vi "ExecuteFile.vi"(0 "File Name With Extension":string) -> ()   [LabVIEW 2015]
panel:
  out "error out":errorcluster
  out "File Contents":string
  out "Lines":string[](array[string])
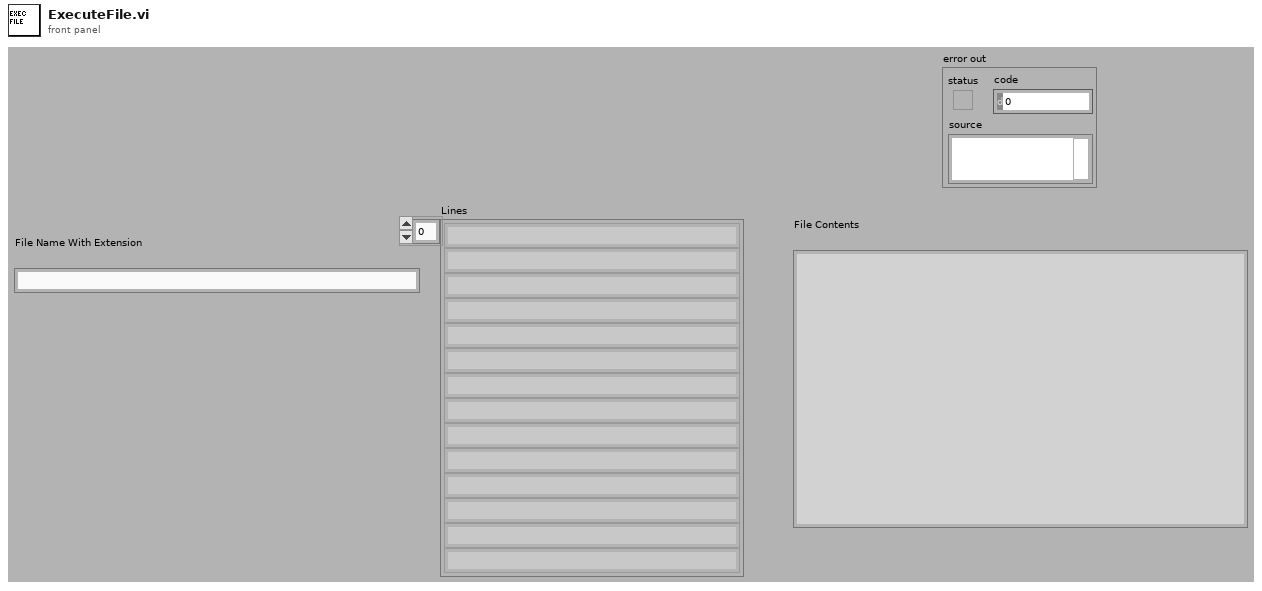
[diagram p1: front panel]
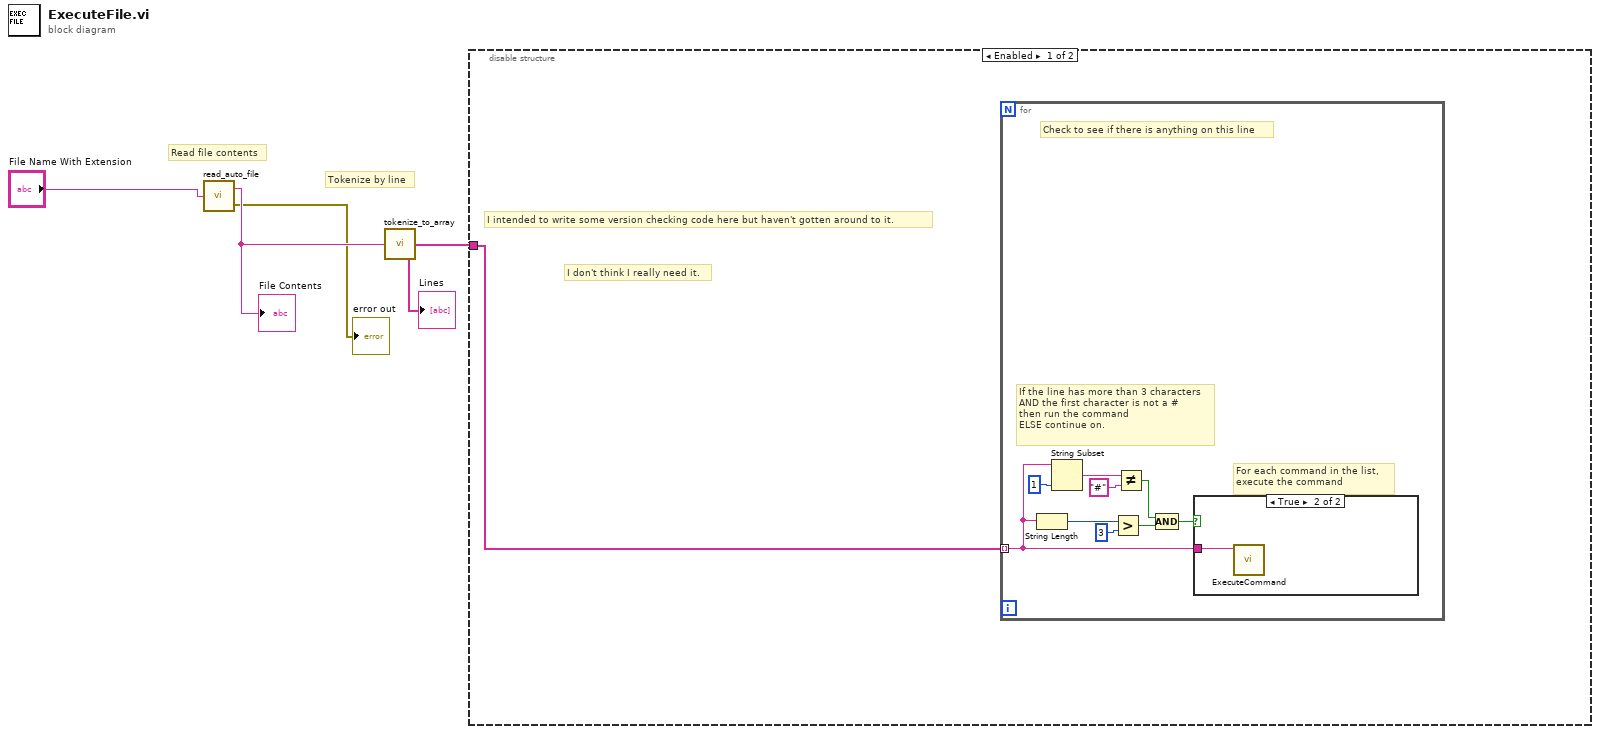
[diagram p0: block diagram]
diagram:
  # "Tokenize by line"
  # "Read file contents"
  n1 = call "read_auto_file.vi"("File Name With Extension"="File Name With Extension") -> ("File Contents"=w4:string, "error out"=→"error out":errorcluster)
  "File Contents" <- w4
  n2 = call "tokenize_to_array.vi"("File Contents"=w4) -> ("Lines"=w2:string[])
  "Lines" <- w2
  n3 = disable-structure shown="Enabled" {
    disable-tunnel: w2 -> [w5 _]
    frame Enabled {
      # "I don't think I really need it."
      # "I intended to write some version checking code here but haven't gotten around to it."
      n4 = for {
        tunnel: w5 -> [w10] mode=indexing
        # "If the line has more than 3 characters\nAND the first character is not a #\nthen run the command\nELSE continue on."
        # "Check to see if there is anything on this line"
        # "For each command in the list,\nexecute the command"
        n5 = String Length(string=w10) -> (length=w14:i32)
        n6 = String Subset(string=w10, length (rest)=1 ("length (rest)")) -> (substring=w8:string)  [unwired: 1 out]
        n7 = Greater?(x=w14, y=3) -> (0:w11:bool)
        n8 = Not Equal?(x=w8, y="#") -> (x != y?=w6:bool)
        n9 = Compound Arithmetic op=AND(w6, w11) -> (w12:bool)
        n10 = case shown="True" w12 {
          tunnel: w10 -> [_ w15]
          frame False {
          }
          frame True {
            n11 = call "ExecuteCommand.vi"("Command"=w15) -> ()  [unwired: 11 out]
          }
        }
      }
    }
    frame Disabled {
    }
  }
